vi "Measured Data Example (B).vi"() -> ()   [LabVIEW 2011]
uses:
  C:/Program Files/Metrohm Autolab/Autolab SDK 1.10/EcoChemie.Autolab.Sdk.dll
  EcoChemie.Autolab.Sdk.dll
panel:
  out "Numeric":i32
  out "Y: EI_0.CalcCurrent":dbl[](array[numeric])
  out "X: SetPointApplied":dbl[](array[numeric])
  out "XY Graph":cluster{"Values":dbl[], "Values":dbl[]}(graph)
  in  "stop":bool
  out "error out":errorcluster
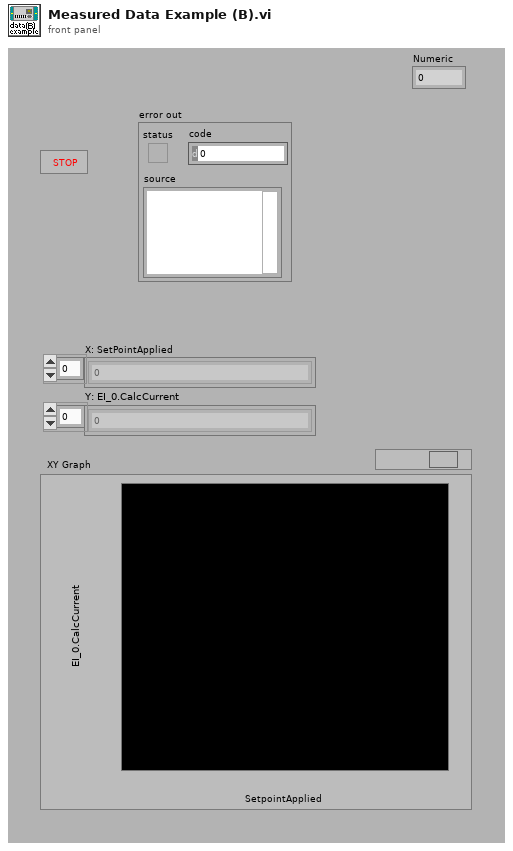
[diagram p1: front panel]
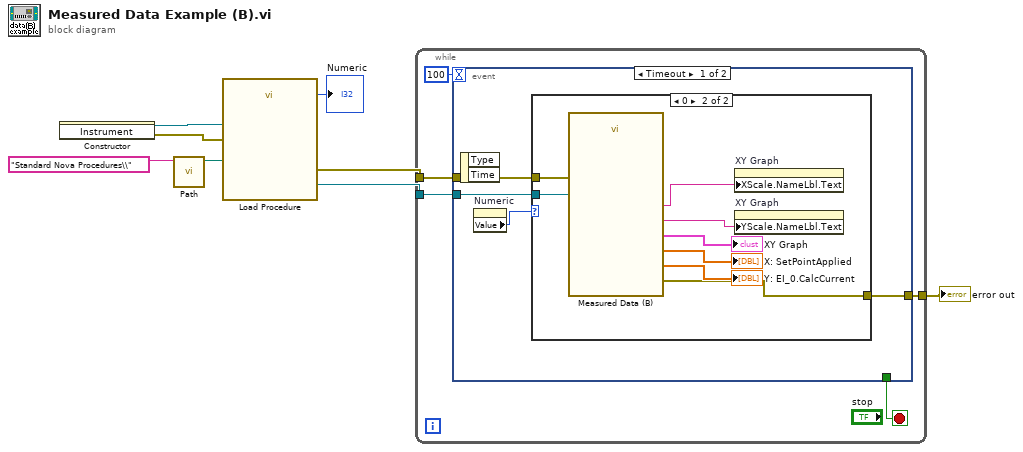
[diagram p0: block diagram]
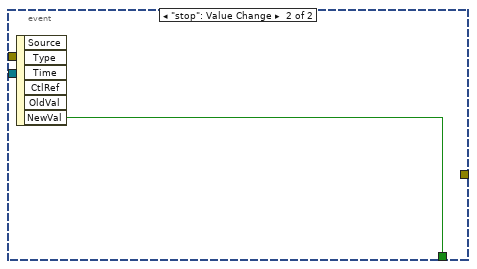
[diagram p3: hidden frame]
diagram:
  n1 = constructor class="Instrument"() -> (reference out=w5:refnum<k24>, error out=w4:errorcluster)  [unwired: 3 in, 1 out]
  n2 = call "Path.vi"("name or relative path"="Standard Nova Procedures\\") -> ("appended path"=w3:path)  [unwired: 10 in]
  n3 = call "Load Procedure.vi"("error in (no error)"=w4, "Procedure"=w3, "Instrument"=w5) -> ("error out"=w7:errorcluster, "Numeric"=→"Numeric":i32, "LoadProcedure"=w6:refnum<k24>)  [unwired: 5 in, 1 out]
  n4 = while {
    tunnel: w7 -> [w13]
    tunnel: w6 -> [w12]
    tunnel: [w11] -> w2
    stop <- w10 stop-if-true
    n5 = event shown="[0] Timeout" {
      selector: _ -> [_ _]
      dyn-events: _ -> [_ _]
      timeout: 100 -> [_ _]
      tunnel: w13 -> [w17 _]
      tunnel: w12 -> [w16 _]
      tunnel: [w15 _] -> w11
      tunnel: [_ w27] -> w10
      event Timeout {
        n6 = event-data() -> ()  [unwired: 1 in, 2 out]
        n7 = property on="Numeric" class="DigNum (strict)"() -> ("Value"=w14:i32)  [unwired: 2 in, 2 out]
        n8 = case shown="0" w14 {
          tunnel: w17 -> [w18 w21]
          tunnel: w16 -> [_ w20]
          tunnel: [w18 w19] -> w15
          frame 2, Default {
          }
          frame 0 {
            n9 = call "Measured Data (B).vi"("LoadProcedure"=w20, "error in (no error)"=w21) -> ("Value X"=→"X: SetPointApplied":dbl[], "Value Y"=→"Y: EI_0.CalcCurrent":dbl[], "Signal X sel"=w22:string, "XY Graph"=→"XY Graph":cluster{"Values":dbl[], "Values":dbl[]}, "Signal Y sel"=w23:string, "error out"=w19:errorcluster)  [unwired: 12 in]
            n10 = property on="XY Graph" class="XYGraph (strict)"("XScale.NameLbl.Text"=w22) -> ()  [unwired: 2 in, 2 out]
            n11 = property on="XY Graph" class="XYGraph (strict)"("YScale.NameLbl.Text"=w23) -> ()  [unwired: 2 in, 2 out]
          }
        }
      }
      event "stop": Value Change {
        n12 = event-data() -> ("NewVal"=w27:bool)  [unwired: 1 in, 5 out]
      }
    }
  }
  "error out" <- w2
